vi "Read Menue 2.vi"(8 "error in (no error)":errorcluster, 11 "MenueItem in":refnum<class "MenueItem.lvclass">) -> (0 "error out":errorcluster, 2 "Menue 2":refnum<user-event>, 3 "MenueItem out":refnum<class "MenueItem.lvclass">)   [LabVIEW 2016, in "MenueItem.lvclass"]
uses:
  MenueItem.lvclass
  MenueItem.lvclass/MenueItem.ctl
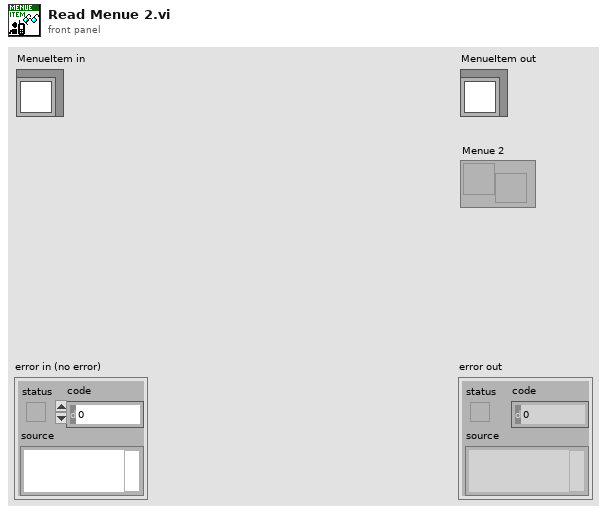
[diagram p1: front panel]
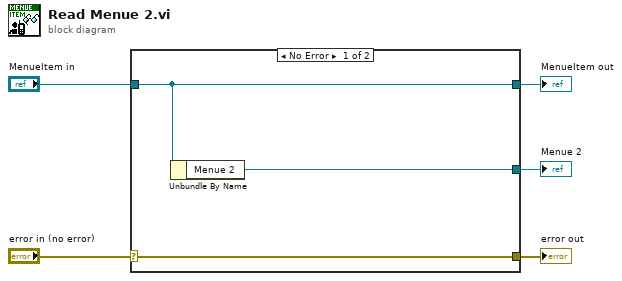
[diagram p0: block diagram]
diagram:
  n1 = case shown="No Error" "error in (no error)" {
    selector: "error in (no error)" -> [w8 w9]
    tunnel: [w8 w9] -> w4
    tunnel: [w7 w10] -> w2
    tunnel: "MenueItem in" -> [w7 w10]
    tunnel: [w6 _] -> w1
    frame No Error {
      n2 = Unbundle By Name(w7) -> ("Menue 2"=w6:refnum<user-event>)
    }
    frame Error {
    }
  }
  "error out" <- w4
  "MenueItem out" <- w2
  "Menue 2" <- w1
